vi "Compute Average.vi"(8 "error in (no error)":errorcluster, 10 "Data":dbl[](array[numeric]), 11 "Video Processor in":refnum<class "Video Processor.lvclass">) -> (0 "error out":errorcluster, 3 "Video Processor out":refnum<class "Video Processor.lvclass">)   [LabVIEW 2018, in "Video Processor.lvclass"]
uses:
  Video Processor.lvclass
  Video Processor.lvclass/Video Processor.ctl
  Roughness Averager/Roughness Averager.lvclass
  C:/Users/aaron.jencks/Documents/GitHub/emerson_seed_object_detection/LabVIEW/Projects/Paul's Video Viewer/Classes/Averager/Averager.lvclass
  C:/Users/aaron.jencks/Documents/GitHub/emerson_seed_object_detection/LabVIEW/Projects/Paul's Video Viewer/Classes/Standard Averager/Standard Averager.lvclass
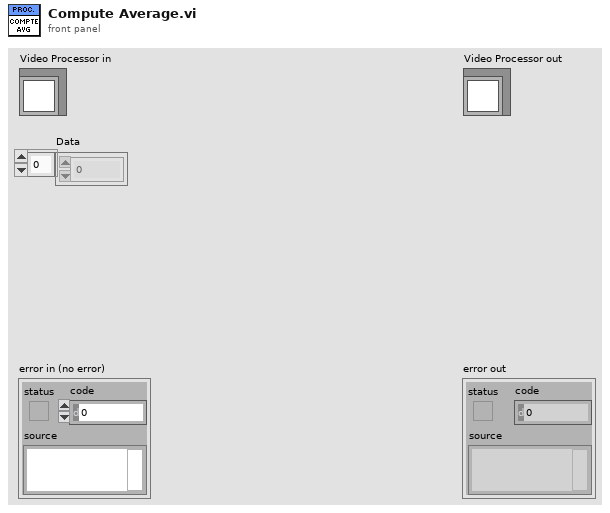
[diagram p1: front panel]
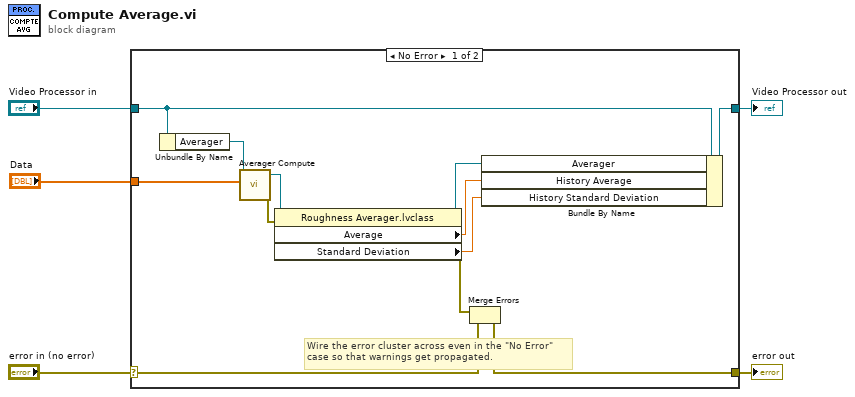
[diagram p0: block diagram]
diagram:
  n1 = case shown="No Error" "error in (no error)" {
    selector: "error in (no error)" -> [w7 w19]
    tunnel: [w6 w19] -> w4
    tunnel: [w10 w18] -> w2
    tunnel: "Video Processor in" -> [w14 w18]
    tunnel: "Data" -> [w16 _]
    frame No Error {
      # "Wire the error cluster across even in the \"No Error\"\ncase so that warnings get propagated."
      n2 = Unbundle By Name(w14) -> ("Averager"=w17:refnum<class "Roughness Averager.lvclass">)
      n3 = call-dynamic "Averager Compute.vi"("Data"=w16, "Roughness Averager in"=w17) -> ("error out"=w9:errorcluster, "Roughness Averager out"=w15:refnum<class "Roughness Averager.lvclass">)  [unwired: 8 in]
      n4 = property class="Roughness Averager.lvclass"(reference=w15, error in=w9) -> (reference out=w11:refnum<class "Roughness Averager.lvclass">, error out=w8:errorcluster, "Average"=w13:dbl, "Standard Deviation"=w12:dbl)
      n5 = Merge Errors(w8, w7) -> (w6:errorcluster)
      n6 = Bundle By Name(cluster=w14, "Averager"=w11, "History Average"=w13, "History Standard Deviation"=w12) -> (w10:refnum<class "Video Processor.lvclass">)
    }
    frame Error {
    }
  }
  "error out" <- w4
  "Video Processor out" <- w2
